vi "plusforlua.vi"(10 "y":dbl, 11 "x":dbl) -> (3 "z":dbl)   [LabVIEW 2011]
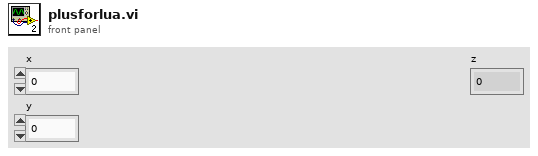
[diagram p1: front panel]
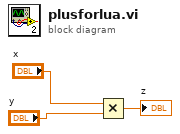
[diagram p0: block diagram]
diagram:
  n1 = Multiply(x="x", y="y") -> (x*y=→"z":dbl)
